vi "lab2(2).vi"() -> ()   [LabVIEW 2024]
uses:
  <vilib>/Analysis/2dsp.llb/Real FFT.vi
  <vilib>/Analysis/3filter.llb/Butterworth Filter (DBL).vi
  <vilib>/Analysis/NI_AALBase.lvlib
  <vilib>/Analysis/NI_AALPro.lvlib
panel:
  out "FFT of filtererd signal":dbl[](graph)
  out "FFT of Noise":dbl[](graph)
  in  "Samples":dbl
  in  "Seed":dbl
  in  "Standard Deviation":dbl(slide) scale=0.0..10.0
  in  "Amplitude":dbl(slide) scale=0.0..10.0
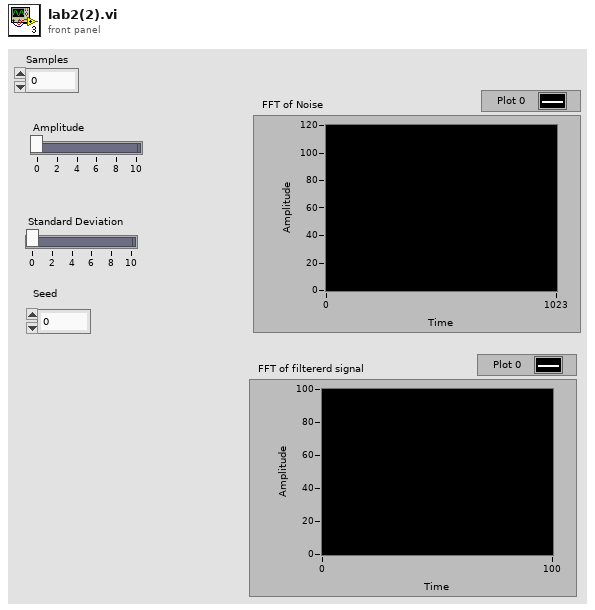
[diagram p1: front panel]
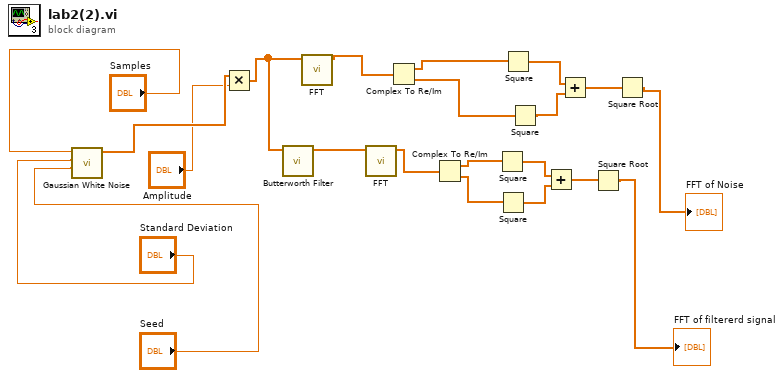
[diagram p0: block diagram]
diagram:
  n1 = call <vilib>:"Gaussian White Noise.vi"("seed"="Seed", "standard deviation"="Standard Deviation", "samples"="Samples") -> ("Gaussian noise pattern"=w18:dbl[])  [unwired: 7 in, 1 out]
  n2 = Multiply(x=w18, y="Amplitude") -> (x*y=w9:dbl[])
  n3 = call-poly <vilib>:"Butterworth Filter.vi"("X"=w9) -> ("Filtered X"=w8:dbl[])  [unwired: 7 in, 1 out]
  n4 = call-poly <vilib>:"FFT.vi"("X"=w9) -> ("FFT {X}"=w11:cdb[])  [unwired: 9 in, 1 out]
  n5 = call-poly <vilib>:"FFT.vi"("X"=w8) -> ("FFT {X}"=w7:cdb[])  [unwired: 9 in, 1 out]
  n6 = Complex To Re/Im(x + iy=w11) -> (x=w16:dbl[], y=w15:dbl[])
  n7 = Complex To Re/Im(x + iy=w7) -> (x=w6:dbl[], y=w5:dbl[])
  n8 = Square(x=w6) -> (x^2=w4:dbl[])
  n9 = Square(x=w5) -> (x^2=w3:dbl[])
  n10 = Square(x=w16) -> (x^2=w14:dbl[])
  n11 = Square(x=w15) -> (x^2=w13:dbl[])
  n12 = Add(x=w4, y=w3) -> (x+y=w2:dbl[])
  n13 = Add(x=w14, y=w13) -> (x+y=w12:dbl[])
  n14 = Square Root(x=w2) -> (sqrt(x)=→"FFT of filtererd signal":dbl[])
  n15 = Square Root(x=w12) -> (sqrt(x)=→"FFT of Noise":dbl[])
